vi "SetupStage.vi"() -> ()   [LabVIEW 2009]
uses:
  StageType.ctt
panel:
  in  "Host address":string="141.84.139.9"
  in  "Case Constant\n(See Context Help)":bool
  in  "error in (no error)":errorcluster
  out "error out":errorcluster
  in  "Stage Setup":bool caption="Analog Setup"
  in  "Stage Type":T1=enum."PI analogue step" caption="Stage Type (input)"
  in  "Analog Setup":bool
  in  "Cancel Button":bool
  in  "OK Button":bool
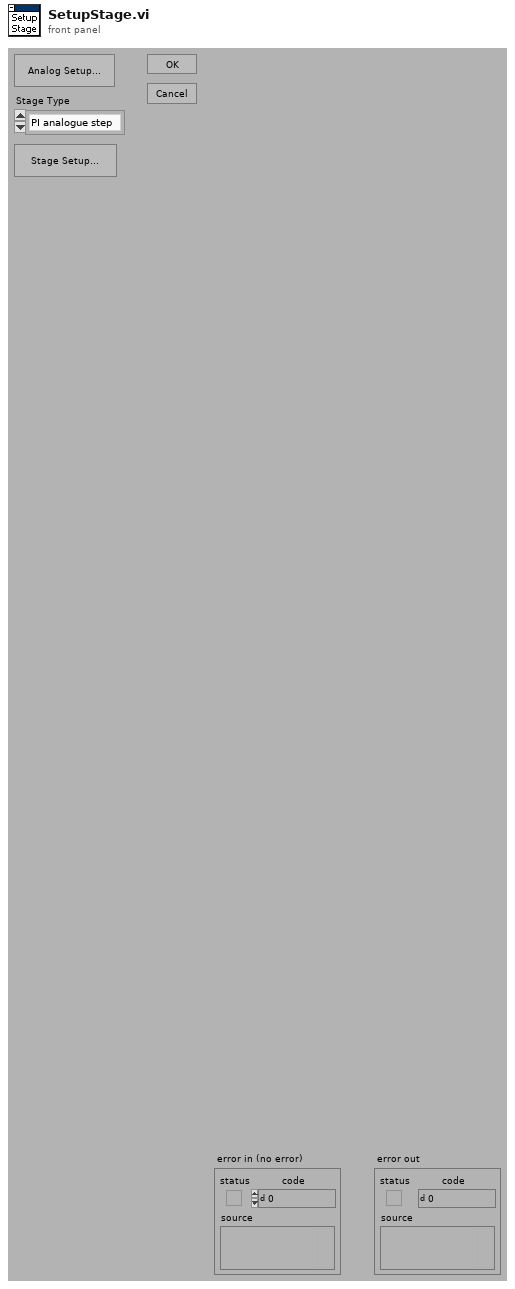
[diagram p1: front panel]
types:
  T1 = typedef "StageType.ctt" = enum16{"PI 725 USB", "PI 725 TCP/IP", "PI analogue step"}
  T2 = enum16{"Get Type", "Set Type", "GetStageInit", "GetWriteStageSetting", "GetInitializeStageOutput", "GetSetAxisPosition", "GetSetPos"}
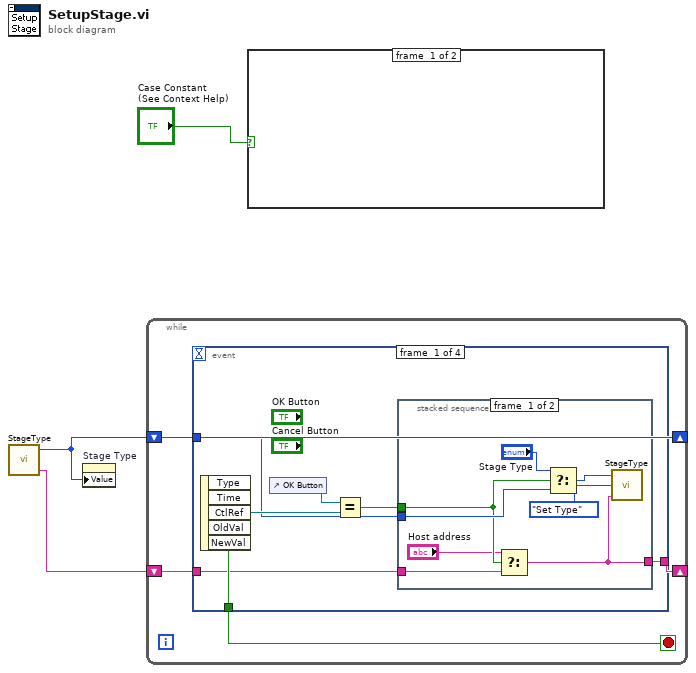
[diagram p0: block diagram]
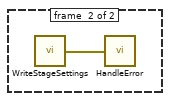
[diagram p3: hidden frame]
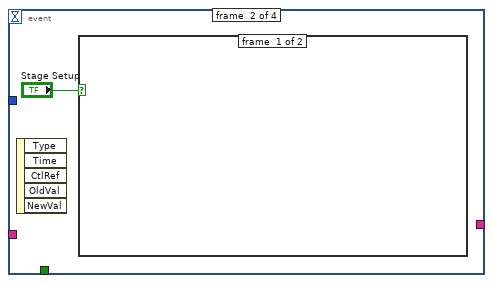
[diagram p4: hidden frame]
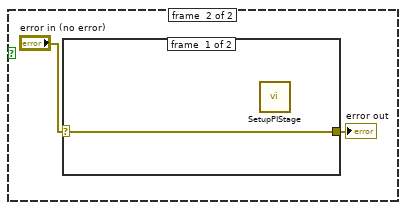
[diagram p5: hidden frame]
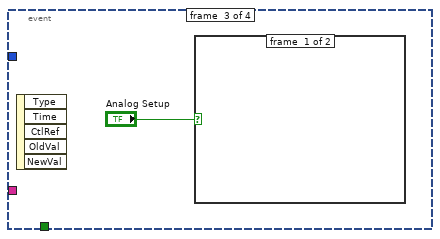
[diagram p7: hidden frame]
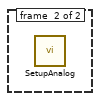
[diagram p8: hidden frame]
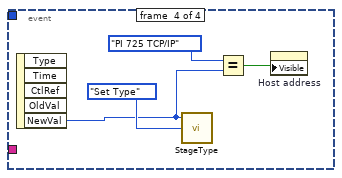
[diagram p9: hidden frame]
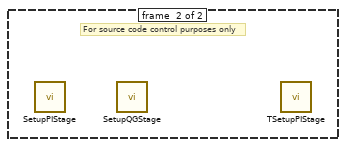
[diagram p10: hidden frame]
diagram:
  n1 = call "StageType.vi"() -> ("Host address (out)"=w1:string, "Stage Type (output)"=w2:T1)  [unwired: 3 in, 1 out]
  n2 = property on="Stage Type" class="Enum (strict)"("Value"=w2) -> ()  [unwired: 2 in, 2 out]
  n3 = while {
    shift-right: [w6] -> _
    shift-left: w2 -> [w6]
    shift-right: [w4] -> _
    shift-left: w1 -> [w5]
    stop <- w7 stop-if-true
    n4 = event shown="[1] \"Stage Setup\": Value Change" {
      selector: _ -> [_ _ _ _]
      dyn-events: _ -> [_ _ _ _]
      timeout: _ -> [_ _ _ _]
      tunnel: [w13 _ _ _] -> w7
      tunnel: w6 -> [w11 _ _ _]
      tunnel: w5 -> [w9 _ _ _]
      tunnel: [w8 _ _ _] -> w4
      event #0 {
        n5 = event-data() -> ("CtlRef"=w14:refnum<vi>, "NewVal"=w13:bool)  [unwired: 1 in, 3 out]
        n6 = control-ref of="OK Button"() -> (w12:refnum<vi>)
        n7 = Equal?(x=w12, y=w14) -> (x = y?=w10:bool)
        n8 = stacked-sequence {
          tunnel: w11 -> [w19 _]
          tunnel: w10 -> [w17 w23]
          tunnel: w9 -> [w18 _]
          tunnel: [w15 _] -> w8
          frame #0 {
            n9 = Select(t="Host address", s=w17, f=w18) -> (s? t:f=w15:string)
            n10 = Select(t="Stage Type", s=w17, f=w19) -> (s? t:f=w21:T1)
            n11 = call "StageType.vi"("Host address"=w15, "Function"=T2."Set Type", "Stage Type (input)"=w21) -> ()  [unwired: 3 out]
          }
          frame #1 {
            n12 = case shown="True" w23 {
              frame #0 {
              }
              frame #1 {
                n13 = call "WriteStageSettings.vi"() -> ("error out"=w24:errorcluster)  [unwired: 1 in]
                n14 = call "HandleError.vi"("error in (no error)"=w24) -> ()
              }
            }
          }
        }
      }
      event #1 {
        n15 = event-data() -> ()  [unwired: 1 in, 5 out]
        n16 = case shown="True" "Stage Setup" {
          frame #0 {
          }
          frame #1 {
            n17 = case shown="No Error" "error in (no error)" {
              selector: "error in (no error)" -> [w28 w29]
              tunnel: [w28 w29] -> w27
              frame #0 {
                n18 = call "SetupPIStage.vi"() -> ()  [unwired: 1 in]
              }
              frame #1 {
              }
            }
            "error out" <- w27
          }
        }
      }
      event #2 {
        n19 = event-data() -> ()  [unwired: 1 in, 5 out]
        n20 = case shown="True" "Analog Setup" {
          frame #0 {
          }
          frame #1 {
            n21 = call "SetupAnalog.vi"() -> ()  [unwired: 1 in]
          }
        }
      }
      event #3 {
        n22 = event-data() -> ("NewVal"=w32:T1)  [unwired: 1 in, 4 out]
        n23 = call "StageType.vi"("Function"=T2."Set Type", "Stage Type (input)"=w32) -> ()  [unwired: 1 in, 3 out]
        n24 = Equal?(x=StageType.ctt."PI 725 TCP/IP", y=w32) -> (x = y?=w33:bool)
        n25 = property on="Host address" class="Str"("Visible"=w33) -> ()  [unwired: 2 in, 2 out]
      }
    }
  }
  n26 = case shown="True" "Case Constant\n(See Context Help)" {
    frame #0 {
    }
    frame #1 {
      # "For source code control purposes only"
      n27 = call "SetupPIStage.vi"() -> ()  [unwired: 1 in]
      n28 = call "SetupQGStage.vi"() -> ()  [unwired: 1 in]
      n29 = call "TSetupPIStage.vi"() -> ()  [unwired: 1 in]
    }
  }
